vi "Enclose with Error Case Structure.vi"(6 "Variant in":variant, 7 "Shift Pressed?":bool, 8 "error in (no error)":errorcluster, 10 "QD Combo Box Ref":refnum<vi>, 11 "QD Launch VI Ref":refnum<vi>) -> (0 "error out":errorcluster, 4 "Variant out":variant)   [LabVIEW 2017]
doc: "Enclose selection with error case structure.\n\nDefault Shortcut - [E]"
uses:
  <vilib>/Utility/error.llb/Error Cluster From Error Code.vi
  <vilib>/ErrorRing/Error Ring.xnode
  <vilib>/Utility/SystemLogging/NI_SystemLogging.lvlib
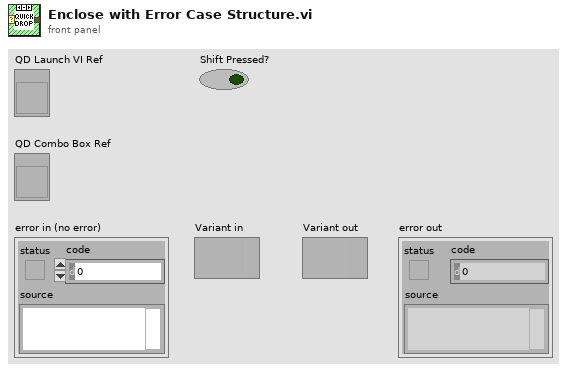
[diagram p1: front panel]
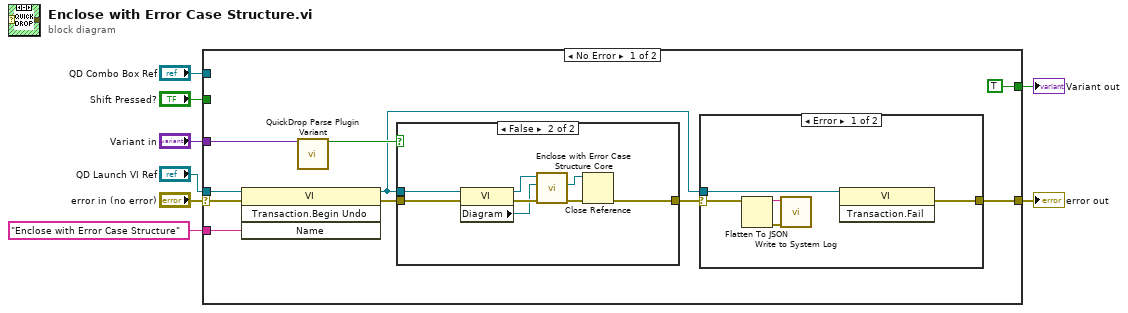
[diagram p0: block diagram]
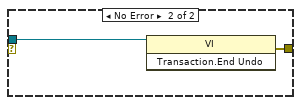
[diagram p2: hidden frame]
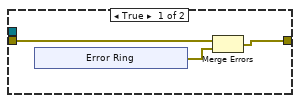
[diagram p3: hidden frame]
diagram:
  n1 = case shown="No Error" "error in (no error)" {
    selector: "error in (no error)" -> [w17 w42]
    tunnel: [w11 w42] -> w2
    tunnel: "QD Launch VI Ref" -> [w16 _]
    tunnel: "Variant in" -> [w18 _]
    tunnel: "Enclose with Error Case Structure" ("Undo Name") -> [w15 _]
    tunnel: [TRUE _] -> w1
    tunnel: "QD Combo Box Ref" -> [_ _]
    tunnel: "Shift Pressed?" -> [_ _]
    frame No Error {
      n2 = invoke class="VI" method="Transaction.Begin Undo"(reference=w16, error in=w17, "Name"=w15) -> (reference out=w10:refnum<vi>, error out=w12:errorcluster)  [unwired: 1 in, 2 out]
      n3 = call <vilib>:"QuickDrop Parse Plugin Variant.vi"("QDKS Variant in"=w18) -> ("QD Launch VI Panel?"=w13:bool)  [unwired: 12 in, 2 out]
      n4 = case shown="False" w13 {
        tunnel: w12 -> [w27 w40]
        tunnel: w10 -> [_ w39]
        tunnel: [w26 w34] -> w9
        frame True {
          n5 = xnode "Error Ring"() -> ("error out"=w28:errorcluster)
          n6 = Merge Errors(w27, w28) -> (w26:errorcluster)
        }
        frame False {
          n7 = property class="VI"(reference=w39, error in=w40) -> (reference out=w38:refnum<vi>, error out=w41:errorcluster, "Diagram"=w37:refnum<vi>)
          n8 = call "Enclose with Error Case Structure Core.vi"("error in (no error)"=w41, "block diagram in"=w37, "VI in"=w38) -> ("error out"=w35:errorcluster, "block diagram out"=w36:refnum<vi>)  [unwired: 6 in, 1 out]
          n9 = Close Reference(reference=w36, error in (no error)=w35) -> (error out=w34:errorcluster)
        }
      }
      n10 = case shown="Error" w9 {
        selector: w9 -> [w21 _]
        tunnel: w10 -> [w22 w24]
        tunnel: [w23 w25] -> w11
        frame Error {
          n11 = Flatten To JSON(anything=w21) -> (JSON string=w20:string, 11:w19:errorcluster)  [unwired: 2 in]
          n12 = call <vilib>:"Write to System Log.vi"("error in (no error)"=w19, "message"=w20) -> ()  [unwired: 9 in, 1 out]
          n13 = invoke class="VI" method="Transaction.Fail"(reference=w22) -> (error out=w23:errorcluster)  [unwired: 2 in, 2 out]
        }
        frame No Error {
          n14 = invoke class="VI" method="Transaction.End Undo"(reference=w24) -> (error out=w25:errorcluster)  [unwired: 2 in, 2 out]
        }
      }
    }
    frame Error {
    }
  }
  "error out" <- w2
  "Variant out" <- w1
